vi "AlliGator Initialize Internal Variables.vi"(8 "error in (no error)":errorcluster, 9 "Alligator version":string, 10 "State Indicators":refnum<vi>, 11 "Graph References":refnum<vi>[](array[refnum])) -> (0 "error out":errorcluster, 1 "Message":string)   [LabVIEW 2021, in "AlliGator Action Engine.lvlib"]
doc: "Initializes AlliGator internal variables."
uses:
  AlliGator Action Engine.lvlib
  AlliGator State Indicators List.ctl
  Globals, Variables, Constants/AlliGator Variables List.ctl
  Image/Image Zoom Factor.ctl
  GUI/AlliGator Skippable Windows Status.ctl
  ROIs/AlliGator ROI Manager Actions.ctl
  Phasor Plot/AlliGator Phasor Harmonic Manager Actions.ctl
  Source Image/AlliGator Displayed Image.ctl
  Local Decay Window/AlliGator Local Decay Fit Results.ctl
  Image Profile Window/AlliGator Image Profile Plot Data.ctl
  Graphs/XY Graph/XY Graph Plot Data.ctl
  Image Profile Window/AlliGator Image Profile Data.ctl
  Image/Image ROI Type.ctl
  Lifetime & Other Parameters/AlliGator Lifetime & Other Parameters Plot Metadata.ctl
  GUI/AlliGator GUI.lvlib
  Globals, Variables, Constants/AlliGator Globals, Variables & Constants.lvlib
  Image/Image.lvlib
  Graphs/XY Graph/XY Graph Add-Ons.lvlib
  ROIs/AlliGator ROIs.lvlib
  Phasor Plot/AlliGator Phasor Plot.lvlib
  Image Profile Window/AlliGator Image Profile Window.lvlib
  Source Image/AlliGator Source Image.lvlib
  Local Decay Window/AlliGator Local Decay Window.lvlib
  Strings/Strings.lvlib
  Phasor Graph/AlliGator Phasor Graph.lvlib
  Lifetime & Other Parameters/AlliGator Lifetime & Other Parameters.lvlib
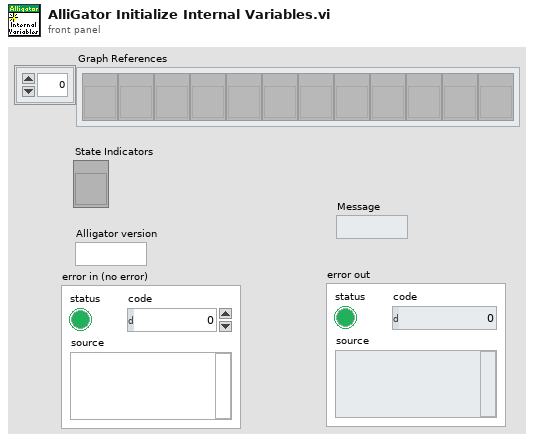
[diagram p1: front panel]
types:
  T1 = typedef "AlliGator Lifetime & Other Parameters.lvlib/AlliGator Lifetime & Other Parameters Plot Metadata.ctl" = cluster{"Intensity Array":dbl[]}
  T2 = typedef "AlliGator Image Profile Window.lvlib/AlliGator Image Profile Data.ctl" = cluster{"ROI Type":T3, "End Points":cluster{"X":dbl, "Y":dbl}[], "Profile Data":T4[]}
  T3 = typedef "Image.lvlib/Image ROI Type.ctl" = enum16{"No Selection", "Point", "Line", "Rectangle", "Oval", "Polygon", "Freehand Region", "Annulus", "Unused2", "Unused3", "Broken Line", "Freehand Line", "Rotated Rectangle"}
  T4 = typedef "AlliGator Image Profile Window.lvlib/AlliGator Image Profile Plot Data.ctl" = cluster{"Plot Name":string, "Plot":T5}
  T5 = typedef "XY Graph Add-Ons.lvlib/XY Graph Plot Data.ctl" = cluster{"X Array":dbl[], "Y Array":dbl[]}
  T6 = typedef "AlliGator Globals, Variables & Constants.lvlib/AlliGator Variables List.ctl" = enum16{"---- GUI ----", "GUI:Initialization Status", "GUI:State Indicators Refnum", "GUI:Original AlliGator Menu Items", "GUI:Current Action Loop State", "GUI:Script in progress", "GUI:Playback", "GUI:Loop Playback", "GUI:Search ROI Used", "GUI:Search ROI", "Decay Graph Max Legend Size", "Intensity Graph Max Legend Size", "Decay Statistics Graph Max Legend Size", "Phasor Graph Max Legend Size", "Phasor Ratio Graph Max Legend Size", "Lifetime Graph Max Legend Size", "---- Files ----", "Files:Export Dataset Frames as Individual Files", "Files:Show Batch Export Help Balloons", "Files:Frames in Dataset", "Files:ptu File Frame Start Indices", "Files:Current Frame in Dataset", "Files:Current Frame Timestamp", "Files:Dataset Loaded", "Files:Dataset Metadata", "Files:Dataset Channel", "Files:Dataset Data Description", "Files:Background Dataset Metadata", "Files:Background Dataset Channel", "Files:Background Dataset Data Description", "Files:Background File Subtraction", "Files:Background File Path", "Files:Background File Pile-up Correction", "Files:Background File Pixel Well Capacity", "Files:Background File Scaling Factor", "Files:Current Dataset Load Settings", "Files:Dataset Path", "Files:ICCD-specific Information", "Files:Macrotime Gate Separation", "------ Python Plugins ------", "Python Plugins:Information", "Python Plugins:Python Session", "Python Plugins:Valid Python Session?", "---- Source Image ----", "Source Image:ROIs", "Source Image:Current ROI", "Source Image:ROI Event Refnum", "X_Source Image:Display Range", "X_Source Image:Palette Information", "X_Source Image:Type of Displayed Image", "X_Time Gate Slider", "Source Image:Palette List", "Source Image:Scale", "Source Image:ROI Overlay Color", "Source Image:Overlay to Erase", "Source Image:Is Displayed Image Accumulated", "Source Image:White Light Image Modified", "Source Image:Mask Image Modified", "---- Image Profile Window ----", "Image Profile:Window Event Refnum", "Image Profile:IntensityType", "Image Profile:Intensity Average Type", "Image Profile:Intensity-weighted SDV", "Image Profile:Box Profile Type", "Image Profile:Window Open", "Image Profile:Plotted Fit Parameter", "------ Phasor Graph -------", "Phasor Graph:Show Line", "---- Phasor Plot ---", "Phasor Plot:Parameters Changed", "Phasor Plot:FLI Dataset Modified since last Calculation", "Phasor Harmonics Data", "Selected Phasor Harmonics", "Phasor Harmonic Manager Event Refnum", "Phasor Plot:ROIs", "Phasor Plot:Current ROI", "Phasor Plot:ROI Event Refnum", "Phasor Plot:Image Reference Points", "Phasor Plot:Computed", "Phasor Plot:Palette Information", "Phasor Plot:Palette List", "Phasor Plot:Phasor Ratio Palette Information", "Phasor Plot:Phasor Ratio Palette List", "Phasor Plot:Image Scale", "Phasor Plot:Image Overlay to Erase", "Phasor Plot:Image Elements to Update", "Phasor Plot:Current Calculation Parameters", "Phasor Plot:Current Calibration Options", "Phasor Plot:Reset Cumulated Phasor Plot", "Phasor Plot:Reference 1", "Phasor Plot:Lifetime Reference 1", "Phasor Plot:Reference 1 Frequency", "Phasor Plot:Reference 2", "Phasor Plot:Lifetime Reference 2", "Phasor Plot:Reference 2 Frequency", "---- Decay Analysis ----", "Number of Selected Decays to Fit", "LS Fit Results", "LAR Fit Results", "BS Fit Results", "Last Decay Max - Min", "Best Fit Parameters", "Best Fit Parameter Names", "Actual Size X", "Actual Size Y", "Binning X", "Binning Y", "Actual # Gates", "Dataset Number", "Gates to...", "Gates Skipped", "Gates to keep", "Gate Step", "Gate Separation", "Reversed Gates", "Pile-up Correction", "Pixel Well Capacity", "Background Subtracted", "Background Subtraction Method", "Background Definition Range", "Background File (deprecated)", "Number of Dataset Accumulated", "Array of Accumulated Dataset Paths", "Do Averaged Datasets", "Destination File Path", "Process Plot Target", "Use 1/D as Phasor Frequency", "---- Decay Fit Parameter Map -----", "Decay Fit Parameter Map:Palette Information", "Decay Fit Parameter Map:Palette List", "Decay Fit Parameter Map:X Resolution", "Decay Fit Parameter Map:Y Resolution", "Decay Fit Parameter Map:Use Decay Fit Result Constraints", "Decay Fit Parameter Map:Decay Fit Result Constraints", "Decay Fit Parameter Map:Decay Fit Result Constraints Applied", "---- Parameter Map ----", "Parameter Map:Palette Information", "Parameter Map:Palette List", "------- Local Decay Window ---------", "Local Decay Graph Window:Event Refnum", "Local Decay Graph Window:Use normalized IRF for convolution", "----- Miscellaneous ----", "Misc:Skippable Dialog Windows Status"}
  T7 = typedef "AlliGator Local Decay Window.lvlib/AlliGator Local Decay Fit Results.ctl" = cluster{"Decay, Fit & Residuals":T4[], "Fit Results":string}
  T8 = typedef "AlliGator Source Image.lvlib/AlliGator Displayed Image.ctl" = enum16{"Single Gate", "Sum of All Gates", "Max of All Gates", "Min of All Gates", "-", "White Ligth Image", "Mask Image"}
  T9 = typedef "AlliGator Phasor Plot.lvlib/AlliGator Phasor Harmonic Manager Actions.ctl" = enum16{"Undefined", "Delete Current Harmonic", "Delete Multiple Harmonics", "Delete All Harmonics", "Swap Harmonics", "Insert Harmonics", "Rename Current Harmonic", "Store New Harmonic", "Store Multiple Harmonics", "Select Next Harmonic", "Select Previous Harmonic", "Update Phasor Harmonic Manager Window"}
  T10 = typedef "AlliGator ROIs.lvlib/AlliGator ROI Manager Actions.ctl" = enum16{"Undefined", "Delete Current ROI", "Delete All Unselected ROIs", "Delete Multiple ROIs", "Delete All ROIs", "Swap ROIs", "Insert ROI", "Update Current ROI Descriptor", "Rename Current ROI", "Store New ROI", "Store Multiple ROIs", "Select Next ROI", "Select Previous ROI", "Find Selected ROI", "Show All ROIs", "Update ROI Manager Window", "Merge All ROIs", "Unmerge ROI", "Set Selected ROI by ID"}
  T11 = typedef "AlliGator GUI.lvlib/AlliGator Skippable Windows Status.ctl" = cluster{"Dialog Window Name":string, "Is skipped":bool}
  T12 = typedef "Image.lvlib/Image Zoom Factor.ctl" = enum16{"Zoom to Fit", "Zoom to Fit (Keep Aspect Ratio)", "Other Zoom Factor"}
  T13 = typedef "AlliGator Action Engine.lvlib/AlliGator State Indicators List.ctl" = enum16{"Phasor Calibration Defined", "Phasor Calibration Series Defined", "Phasor Calibration Map Defined", "Phasor Reference 1 Defined", "Phasor Reference 2 Defined", "Lifetime Reference 1 Defined", "Lifetime Reference 2 Defined", "Phasor Calibration Used", "Phasor Calibration Series Used", "Phasor Calibration Map Used", "Dataset Update Needed", "Phasor Plot Update Needed", "Reference/IRF Defined", "Individual IRFs Defined"}
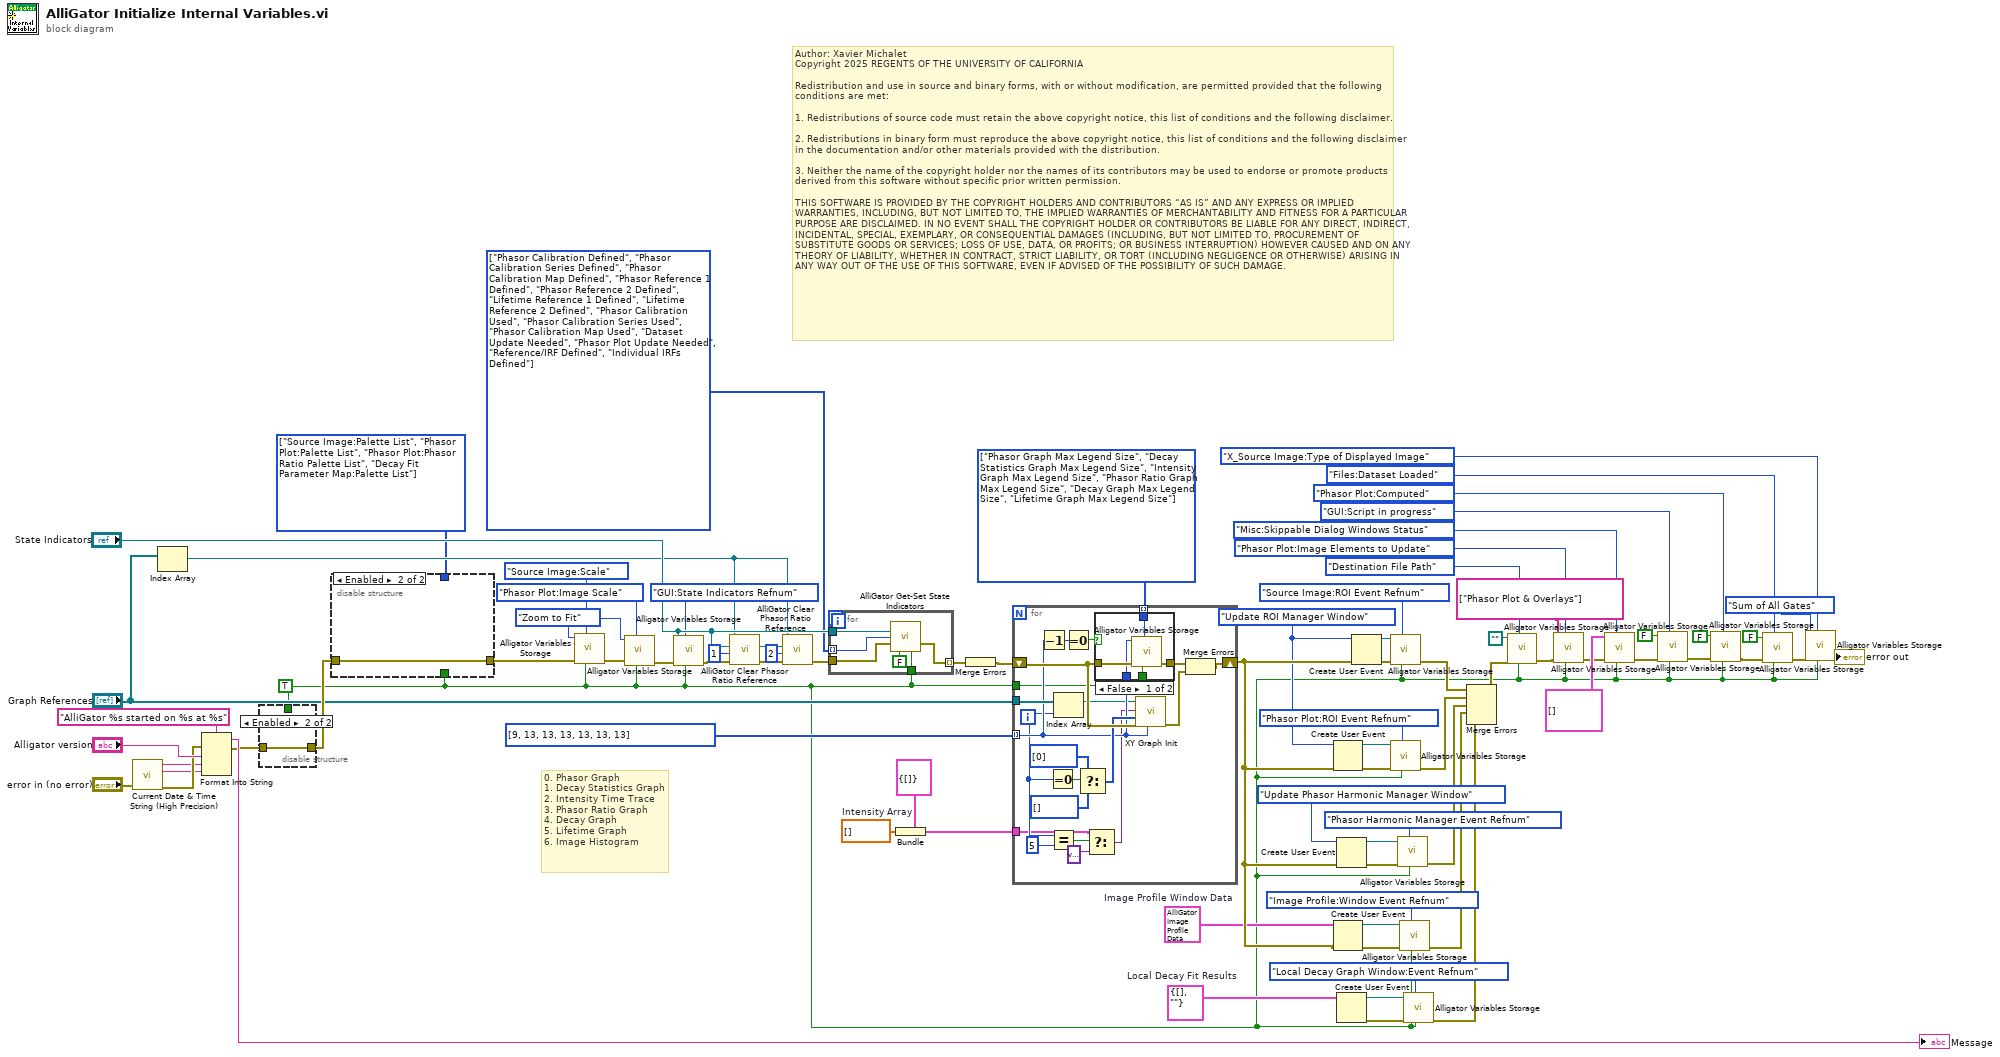
[diagram p0: block diagram]
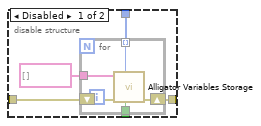
[diagram p2: hidden frame]
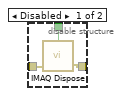
[diagram p3: hidden frame]
diagram:
  w3 = dbl[] []  # Intensity Array
  w6 = T2 {"ROI Type"=enum."No Selection", "End Points"=[{"X"=98.0, "Y"=43.0}, {"X"=133.0, "Y"=78.0}], "Profile Data"=[]}  # Image Profile Window Data
  w8 = T6[] [enum."Source Image:Palette List", enum."Phasor Plot:Palette List", enum."Phasor Plot:Phasor Ratio Palette List", enum."Decay Fit Parameter Map:Palette List"] items=["---- GUI ----", "GUI:Initialization Status", "GUI:State Indicators Refnum", "GUI:Original AlliGator Menu Items", "GUI:Current Action Loop State", "GUI:Script in progress", "GUI:Playback", "GUI:Loop Playback", "GUI:Search ROI Used", "GUI:Search ROI", "Decay Graph Max Legend Size", "Intensity Graph Max Legend Size", "Decay Statistics Graph Max Legend Size", "Phasor Graph Max Legend Size", "Phasor Ratio Graph Max Legend Size", "Lifetime Graph Max Legend Size", "---- Files ----", "Files:Export Dataset Frames as Individual Files", "Files:Show Batch Export Help Balloons", "Files:Frames in Dataset", "Files:ptu File Frame Start Indices", "Files:Current Frame in Dataset", "Files:Current Frame Timestamp", "Files:Dataset Loaded", "Files:Dataset Metadata", "Files:Dataset Channel", "Files:Dataset Data Description", "Files:Background Dataset Metadata", "Files:Background Dataset Channel", "Files:Background Dataset Data Description", "Files:Background File Subtraction", "Files:Background File Path", "Files:Background File Pile-up Correction", "Files:Background File Pixel Well Capacity", "Files:Background File Scaling Factor", "Files:Current Dataset Load Settings", "Files:Dataset Path", "Files:ICCD-specific Information", "Files:Macrotime Gate Separation", "------ Python Plugins ------", "Python Plugins:Information", "Python Plugins:Python Session", "Python Plugins:Valid Python Session?", "---- Source Image ----", "Source Image:ROIs", "Source Image:Current ROI", "Source Image:ROI Event Refnum", "X_Source Image:Display Range", "X_Source Image:Palette Information", "X_Source Image:Type of Displayed Image", "X_Time Gate Slider", "Source Image:Palette List", "Source Image:Scale", "Source Image:ROI Overlay Color", "Source Image:Overlay to Erase", "Source Image:Is Displayed Image Accumulated", "Source Image:White Light Image Modified", "Source Image:Mask Image Modified", "---- Image Profile Window ----", "Image Profile:Window Event Refnum", "Image Profile:IntensityType", "Image Profile:Intensity Average Type", "Image Profile:Intensity-weighted SDV", "Image Profile:Box Profile Type", "Image Profile:Window Open", "Image Profile:Plotted Fit Parameter", "------ Phasor Graph -------", "Phasor Graph:Show Line", "---- Phasor Plot ---", "Phasor Plot:Parameters Changed", "Phasor Plot:FLI Dataset Modified since last Calculation", "Phasor Harmonics Data", "Selected Phasor Harmonics", "Phasor Harmonic Manager Event Refnum", "Phasor Plot:ROIs", "Phasor Plot:Current ROI", "Phasor Plot:ROI Event Refnum", "Phasor Plot:Image Reference Points", "Phasor Plot:Computed", "Phasor Plot:Palette Information", "Phasor Plot:Palette List", "Phasor Plot:Phasor Ratio Palette Information", "Phasor Plot:Phasor Ratio Palette List", "Phasor Plot:Image Scale", "Phasor Plot:Image Overlay to Erase", "Phasor Plot:Image Elements to Update", "Phasor Plot:Current Calculation Parameters", "Phasor Plot:Current Calibration Options", "Phasor Plot:Reset Cumulated Phasor Plot", "Phasor Plot:Reference 1", "Phasor Plot:Lifetime Reference 1", "Phasor Plot:Reference 1 Frequency", "Phasor Plot:Reference 2", "Phasor Plot:Lifetime Reference 2", "Phasor Plot:Reference 2 Frequency", "---- Decay Analysis ----", "Number of Selected Decays to Fit", "LS Fit Results", "LAR Fit Results", "BS Fit Results", "Last Decay Max - Min", "Best Fit Parameters", "Best Fit Parameter Names", "Actual Size X", "Actual Size Y", "Binning X", "Binning Y", "Actual # Gates", "Dataset Number", "Gates to...", "Gates Skipped", "Gates to keep", "Gate Step", "Gate Separation", "Reversed Gates", "Pile-up Correction", "Pixel Well Capacity", "Background Subtracted", "Background Subtraction Method", "Background Definition Range", "Background File (deprecated)", "Number of Dataset Accumulated", "Array of Accumulated Dataset Paths", "Do Averaged Datasets", "Destination File Path", "Process Plot Target", "Use 1/D as Phasor Frequency", "---- Decay Fit Parameter Map -----", "Decay Fit Parameter Map:Palette Information", "Decay Fit Parameter Map:Palette List", "Decay Fit Parameter Map:X Resolution", "Decay Fit Parameter Map:Y Resolution", "Decay Fit Parameter Map:Use Decay Fit Result Constraints", "Decay Fit Parameter Map:Decay Fit Result Constraints", "Decay Fit Parameter Map:Decay Fit Result Constraints Applied", "---- Parameter Map ----", "Parameter Map:Palette Information", "Parameter Map:Palette List", "------- Local Decay Window ---------", "Local Decay Graph Window:Event Refnum", "Local Decay Graph Window:Use normalized IRF for convolution", "----- Miscellaneous ----", "Misc:Skippable Dialog Windows Status"] ("Array")
  w67 = T7 {"Decay, Fit & Residuals"=[], "Fit Results"=""}  # Local Decay Fit Results
  w49 = AlliGator_ROI_Manager_Actions."Update ROI Manager Window" ("Action")
  w20 = T6[] [enum."Phasor Graph Max Legend Size", enum."Decay Statistics Graph Max Legend Size", enum."Intensity Graph Max Legend Size", enum."Phasor Ratio Graph Max Legend Size", enum."Decay Graph Max Legend Size", enum."Lifetime Graph Max Legend Size"] items=["---- GUI ----", "GUI:Initialization Status", "GUI:State Indicators Refnum", "GUI:Original AlliGator Menu Items", "GUI:Current Action Loop State", "GUI:Script in progress", "GUI:Playback", "GUI:Loop Playback", "GUI:Search ROI Used", "GUI:Search ROI", "Decay Graph Max Legend Size", "Intensity Graph Max Legend Size", "Decay Statistics Graph Max Legend Size", "Phasor Graph Max Legend Size", "Phasor Ratio Graph Max Legend Size", "Lifetime Graph Max Legend Size", "---- Files ----", "Files:Export Dataset Frames as Individual Files", "Files:Show Batch Export Help Balloons", "Files:Frames in Dataset", "Files:ptu File Frame Start Indices", "Files:Current Frame in Dataset", "Files:Current Frame Timestamp", "Files:Dataset Loaded", "Files:Dataset Metadata", "Files:Dataset Channel", "Files:Dataset Data Description", "Files:Background Dataset Metadata", "Files:Background Dataset Channel", "Files:Background Dataset Data Description", "Files:Background File Subtraction", "Files:Background File Path", "Files:Background File Pile-up Correction", "Files:Background File Pixel Well Capacity", "Files:Background File Scaling Factor", "Files:Current Dataset Load Settings", "Files:Dataset Path", "Files:ICCD-specific Information", "Files:Macrotime Gate Separation", "------ Python Plugins ------", "Python Plugins:Information", "Python Plugins:Python Session", "Python Plugins:Valid Python Session?", "---- Source Image ----", "Source Image:ROIs", "Source Image:Current ROI", "Source Image:ROI Event Refnum", "X_Source Image:Display Range", "X_Source Image:Palette Information", "X_Source Image:Type of Displayed Image", "X_Time Gate Slider", "Source Image:Palette List", "Source Image:Scale", "Source Image:ROI Overlay Color", "Source Image:Overlay to Erase", "Source Image:Is Displayed Image Accumulated", "Source Image:White Light Image Modified", "Source Image:Mask Image Modified", "---- Image Profile Window ----", "Image Profile:Window Event Refnum", "Image Profile:IntensityType", "Image Profile:Intensity Average Type", "Image Profile:Intensity-weighted SDV", "Image Profile:Box Profile Type", "Image Profile:Window Open", "Image Profile:Plotted Fit Parameter", "------ Phasor Graph -------", "Phasor Graph:Show Line", "---- Phasor Plot ---", "Phasor Plot:Parameters Changed", "Phasor Plot:FLI Dataset Modified since last Calculation", "Phasor Harmonics Data", "Selected Phasor Harmonics", "Phasor Harmonic Manager Event Refnum", "Phasor Plot:ROIs", "Phasor Plot:Current ROI", "Phasor Plot:ROI Event Refnum", "Phasor Plot:Image Reference Points", "Phasor Plot:Computed", "Phasor Plot:Palette Information", "Phasor Plot:Palette List", "Phasor Plot:Phasor Ratio Palette Information", "Phasor Plot:Phasor Ratio Palette List", "Phasor Plot:Image Scale", "Phasor Plot:Image Overlay to Erase", "Phasor Plot:Image Elements to Update", "Phasor Plot:Current Calculation Parameters", "Phasor Plot:Current Calibration Options", "Phasor Plot:Reset Cumulated Phasor Plot", "Phasor Plot:Reference 1", "Phasor Plot:Lifetime Reference 1", "Phasor Plot:Reference 1 Frequency", "Phasor Plot:Reference 2", "Phasor Plot:Lifetime Reference 2", "Phasor Plot:Reference 2 Frequency", "---- Decay Analysis ----", "Number of Selected Decays to Fit", "LS Fit Results", "LAR Fit Results", "BS Fit Results", "Last Decay Max - Min", "Best Fit Parameters", "Best Fit Parameter Names", "Actual Size X", "Actual Size Y", "Binning X", "Binning Y", "Actual # Gates", "Dataset Number", "Gates to...", "Gates Skipped", "Gates to keep", "Gate Step", "Gate Separation", "Reversed Gates", "Pile-up Correction", "Pixel Well Capacity", "Background Subtracted", "Background Subtraction Method", "Background Definition Range", "Background File (deprecated)", "Number of Dataset Accumulated", "Array of Accumulated Dataset Paths", "Do Averaged Datasets", "Destination File Path", "Process Plot Target", "Use 1/D as Phasor Frequency", "---- Decay Fit Parameter Map -----", "Decay Fit Parameter Map:Palette Information", "Decay Fit Parameter Map:Palette List", "Decay Fit Parameter Map:X Resolution", "Decay Fit Parameter Map:Y Resolution", "Decay Fit Parameter Map:Use Decay Fit Result Constraints", "Decay Fit Parameter Map:Decay Fit Result Constraints", "Decay Fit Parameter Map:Decay Fit Result Constraints Applied", "---- Parameter Map ----", "Parameter Map:Palette Information", "Parameter Map:Palette List", "------- Local Decay Window ---------", "Local Decay Graph Window:Event Refnum", "Local Decay Graph Window:Use normalized IRF for convolution", "----- Miscellaneous ----", "Misc:Skippable Dialog Windows Status"] ("Array")
  w18 = Image_Zoom_Factor."Zoom to Fit" ("Image Zoom Factor")
  w5 = TRUE ("Get(F)/Set")
  w15 = T13[] [enum."Phasor Calibration Defined", enum."Phasor Calibration Series Defined", enum."Phasor Calibration Map Defined", enum."Phasor Reference 1 Defined", enum."Phasor Reference 2 Defined", enum."Lifetime Reference 1 Defined", enum."Lifetime Reference 2 Defined", enum."Phasor Calibration Used", enum."Phasor Calibration Series Used", enum."Phasor Calibration Map Used", enum."Dataset Update Needed", enum."Phasor Plot Update Needed", enum."Reference/IRF Defined", enum."Individual IRFs Defined"] items=["Phasor Calibration Defined", "Phasor Calibration Series Defined", "Phasor Calibration Map Defined", "Phasor Reference 1 Defined", "Phasor Reference 2 Defined", "Lifetime Reference 1 Defined", "Lifetime Reference 2 Defined", "Phasor Calibration Used", "Phasor Calibration Series Used", "Phasor Calibration Map Used", "Dataset Update Needed", "Phasor Plot Update Needed", "Reference/IRF Defined", "Individual IRFs Defined"] ("Array")
  # "Author: Xavier Michalet\nCopyright 2025 REGENTS OF THE UNIVERSITY OF CALIFORNIA\n\nRedistribution and use in source and binary forms, with or without modification, are permitted provided that the following conditions are met:\n\n1. Redistributions of source code must retain the above copyright notice, this list of conditions and the following disclaimer.\n\n2. Redistributions in binary form must reproduce the above copyright notice, this list of conditions and the following disclaimer in the documentation and/or other materials provided with the distribution.\n\n3. Neither the name of the copyright holder nor the names of its contributors may be used to endorse or promote products derived from this software without specific prior written permission.\n\nTHIS SOFTWARE IS PROVIDED BY THE COPYRIGHT HOLDERS AND CONTRIBUTORS “AS IS” AND ANY EXPRESS OR IMPLIED WARRANTIES, INCLUDING, BUT NOT LIMITED TO, THE IMPLIED WARRANTIES OF MERCHANTABILITY AND FITNESS FOR A PARTICULAR PURPOSE ARE DISCLAIMED. IN NO EVENT SHALL THE COPYRIGHT HOLDER OR CONTRIBUTORS BE LIABLE FOR ANY DIRECT, INDIRECT, INCIDENTAL, SPECIAL, EXEMPLARY, OR CONSEQUENTIAL DAMAGES (INCLUDING, BUT NOT LIMITED TO, PROCUREMENT OF SUBSTITUTE GOODS OR SERVICES; LOSS OF USE, DATA, OR PROFITS; OR BUSINESS INTERRUPTION) HOWEVER CAUSED AND ON ANY THEORY OF LIABILITY, WHETHER IN CONTRACT, STRICT LIABILITY, OR TORT (INCLUDING NEGLIGENCE OR OTHERWISE) ARISING IN ANY WAY OUT OF THE USE OF THIS SOFTWARE, EVEN IF ADVISED OF THE POSSIBILITY OF SUCH DAMAGE."
  # "0. Phasor Graph\n1. Decay Statistics Graph\n2. Intensity Time Trace\n3. Phasor Ratio Graph\n4. Decay Graph\n5. Lifetime Graph\n6. Image Histogram"
  n1 = call "Current Date & Time String (High Precision).vi"("Error In"="error in (no error)") -> ("Error Out"=w73:errorcluster, "time string"=w72:string, "date string"=w71:string)  [unwired: 7 in, 1 out]
  n2 = Index Array(array="Graph References") -> (element=w13:refnum<vi>)  [unwired: 1 in]
  n3 = Format Into String(format string="AlliGator %s started on %s at %s" ("initial string"), error in=w73, "Alligator version", w71, w72) -> (resulting string=→"Message":string, error out=w9:errorcluster)  [unwired: 1 in]
  n4 = disable-structure shown="Enabled" {
    disable-tunnel: [w84 w85] -> w80
    disable-tunnel: w5 -> [w83 _]
    disable-tunnel: w9 -> [w82 w85]
    frame Disabled {
      n5 = call "IMAQ Dispose"("All Images? (No)"=w83, "error in (no error)"=w82) -> ("error out"=w84:errorcluster)  [unwired: 4 in]
    }
    frame Enabled {
    }
  }
  n6 = disable-structure shown="Enabled" {
    disable-tunnel: w5 -> [w90 _]
    disable-tunnel: w80 -> [w89 w96]
    disable-tunnel: w8 -> [w87 _]
    disable-tunnel: [w86 w96] -> w7
    frame Disabled {
      n7 = for {
        tunnel: w90 -> [w95]
        tunnel: string[] [] ("String Array") -> [w93]
        tunnel: w87 -> [w92] mode=indexing
        shift-right: [w91] -> w86
        shift-left: w89 -> [w94]
        n8 = call "Alligator Variables Storage.vi"("Get(F)/Set"=w95, "AlliGator Variable"=w92, "Error In"=w94, "Data in"=w93) -> ("Error Out"=w91:errorcluster)  [unwired: 5 in, 2 out]
      }
    }
    frame Enabled {
    }
  }
  n9 = call "Alligator Variables Storage.vi"("Get(F)/Set"=w5, "AlliGator Variable"=AlliGator_Variables_List."Source Image:Scale" ("Alligator Variable"), "Error In"=w7, "Data in"=w18) -> ("Error Out"=w17:errorcluster)  [unwired: 5 in, 2 out]
  n10 = call "Alligator Variables Storage.vi"("Get(F)/Set"=w5, "AlliGator Variable"=AlliGator_Variables_List."Phasor Plot:Image Scale" ("Alligator Variable"), "Error In"=w17, "Data in"=w18) -> ("Error Out"=w81:errorcluster)  [unwired: 5 in, 2 out]
  n11 = call "Alligator Variables Storage.vi"("Get(F)/Set"=w5, "AlliGator Variable"=AlliGator_Variables_List."GUI:State Indicators Refnum" ("Alligator Variable"), "Error In"=w81, "Data in"="State Indicators") -> ("Error Out"=w75:errorcluster)  [unwired: 5 in, 2 out]
  n12 = call "AlliGator Clear Phasor Ratio Reference.vi"("error in (no error)"=w75, "Reference Number"=1, "State Indicators Refnum"="State Indicators", "Phasor Graph Refnum"=w13) -> ("Error Out"=w76:errorcluster)  [unwired: 7 in]
  n13 = call "AlliGator Clear Phasor Ratio Reference.vi"("error in (no error)"=w76, "Reference Number"=2, "State Indicators Refnum"="State Indicators", "Phasor Graph Refnum"=w13) -> ("Error Out"=w11:errorcluster)  [unwired: 7 in]
  n14 = for {
    tunnel: "State Indicators" -> [w102]
    tunnel: w15 -> [w101] mode=indexing
    tunnel: w11 -> [w99]
    tunnel: [w98] -> w68 mode=indexing
    tunnel: w5 -> [w97]
    n15 = call "AlliGator Get-Set State Indicators.vi"("State Indicators Refnum"=w102, "AlliGator State Indicators List"=w101, "Error In"=w99, "ON/OFF"=FALSE ("Set (T)/Unset (F)"), "Set (T)/Get"=w97) -> ("Error Out"=w98:errorcluster)  [unwired: 8 in, 2 out]
  }
  n16 = Bundle(cluster=T1 {"Intensity Array"=[]}, "Intensity Array"=w3) -> (w2:T1)
  n17 = Merge Errors(w68) -> (w12:errorcluster)
  n18 = for {
    tunnel: w20 -> [w123] mode=indexing
    tunnel: w5 -> [w109]
    shift-right: [w119] -> w58
    shift-left: w12 -> [w120]
    tunnel: i32[] [9, 13, 13, 13, 13, 13, 13] ("Max Legend Size (8)") -> [w113] mode=indexing
    tunnel: "Graph References" -> [w121]
    tunnel: w2 -> [w105]
    i -> [w108]
    n19 = Decrement(x=w113) -> (x-1=w112:i32)
    n20 = Equal To 0?(x=w108) -> (x = 0?=w117:bool)
    n21 = Equal?(x=w108, y=5) -> (x = y?=w106:bool)
    n22 = Index Array(array=w121, index=w108) -> (element=w110:refnum<vi>)
    n23 = Equal To 0?(x=w112) -> (x = 0?=w111:bool)
    n24 = Select(t=i32[] [0] ("Plots to Skip (none)"), s=w117, f=i32[] []) -> (s? t:f=w116:i32[])
    n25 = Select(t=w105, s=w106, f=variant) -> (s? t:f=w103:variant)
    n26 = case shown="False" w111 {
      tunnel: w123 -> [w128 _]
      tunnel: [w127 w129] -> w122
      tunnel: w120 -> [w126 w129]
      tunnel: w113 -> [w125 _]
      tunnel: w109 -> [w124 _]
      frame False {
        n27 = call "Alligator Variables Storage.vi"("Get(F)/Set"=w124, "AlliGator Variable"=w128, "Error In"=w126, "Data in"=w125) -> ("Error Out"=w127:errorcluster)  [unwired: 5 in, 2 out]
      }
      frame True {
      }
    }
    n28 = call "XY Graph Init.vi"("Max Legend Size (8)"=w113, "Error In"=w120, "Plots to Skip (none)"=w116, "Metadata Type"=w103, "XYGraph in"=w110) -> ("Error Out"=w118:errorcluster)  [unwired: 6 in]
    n29 = Merge Errors(w122, w118) -> (w119:errorcluster)
  }
  n30 = Create User Event(user event datatype=w49, error in=w58) -> (user event=w45:refnum<user-event>, error out=w44:errorcluster)
  n31 = Create User Event(user event datatype=w6, error in=w58) -> (user event=w4:refnum<user-event>, error out=w55:errorcluster)
  n32 = Create User Event(user event datatype=AlliGator_Phasor_Harmonic_Manager_Actions."Update Phasor Harmonic Manager Window" ("Action"), error in=w58) -> (user event=w52:refnum<user-event>, error out=w51:errorcluster)
  n33 = Create User Event(user event datatype=w67) -> (user event=w64:refnum<user-event>, error out=w65:errorcluster)  [unwired: 1 in]
  n34 = Create User Event(user event datatype=w49, error in=w58) -> (user event=w22:refnum<user-event>, error out=w23:errorcluster)
  n35 = call "Alligator Variables Storage.vi"("Get(F)/Set"=w5, "AlliGator Variable"=AlliGator_Variables_List."Source Image:ROI Event Refnum" ("Alligator Variable"), "Error In"=w23, "Data in"=w22) -> ("Error Out"=w24:errorcluster)  [unwired: 5 in, 2 out]
  n36 = call "Alligator Variables Storage.vi"("Get(F)/Set"=w5, "AlliGator Variable"=AlliGator_Variables_List."Phasor Plot:ROI Event Refnum" ("Alligator Variable"), "Error In"=w44, "Data in"=w45) -> ("Error Out"=w47:errorcluster)  [unwired: 5 in, 2 out]
  n37 = call "Alligator Variables Storage.vi"("Get(F)/Set"=w5, "AlliGator Variable"=AlliGator_Variables_List."Phasor Harmonic Manager Event Refnum" ("Alligator Variable"), "Error In"=w51, "Data in"=w52) -> ("Error Out"=w53:errorcluster)  [unwired: 5 in, 2 out]
  n38 = call "Alligator Variables Storage.vi"("Get(F)/Set"=w5, "AlliGator Variable"=AlliGator_Variables_List."Image Profile:Window Event Refnum" ("Alligator Variable"), "Error In"=w55, "Data in"=w4) -> ("Error Out"=w57:errorcluster)  [unwired: 5 in, 2 out]
  n39 = call "Alligator Variables Storage.vi"("Get(F)/Set"=w5, "AlliGator Variable"=AlliGator_Variables_List."Local Decay Graph Window:Event Refnum" ("Alligator Variable"), "Error In"=w65, "Data in"=w64) -> ("Error Out"=w66:errorcluster)  [unwired: 5 in, 2 out]
  n40 = Merge Errors(w24, w47, w53, w57, w66) -> (w46:errorcluster)
  n41 = call "Alligator Variables Storage.vi"("Get(F)/Set"=w5, "AlliGator Variable"=AlliGator_Variables_List."Destination File Path" ("Alligator Variable"), "Error In"=w46, "Data in"=path "") -> ("Error Out"=w27:errorcluster)  [unwired: 5 in, 2 out]
  n42 = call "Alligator Variables Storage.vi"("Get(F)/Set"=w5, "AlliGator Variable"=AlliGator_Variables_List."Phasor Plot:Image Elements to Update" ("Alligator Variable"), "Error In"=w27, "Data in"=string[] ["Phasor Plot & Overlays"] ("element")) -> ("Error Out"=w31:errorcluster)  [unwired: 5 in, 2 out]
  n43 = call "Alligator Variables Storage.vi"("Get(F)/Set"=w5, "AlliGator Variable"=AlliGator_Variables_List."Misc:Skippable Dialog Windows Status" ("Alligator Variable"), "Error In"=w31, "Data in"=T11[] []) -> ("Error Out"=w34:errorcluster)  [unwired: 5 in, 2 out]
  n44 = call "Alligator Variables Storage.vi"("Get(F)/Set"=w5, "AlliGator Variable"=AlliGator_Variables_List."GUI:Script in progress" ("Alligator Variable"), "Error In"=w34, "Data in"=FALSE ("Get(F)/Set")) -> ("Error Out"=w38:errorcluster)  [unwired: 5 in, 2 out]
  n45 = call "Alligator Variables Storage.vi"("Get(F)/Set"=w5, "AlliGator Variable"=AlliGator_Variables_List."Phasor Plot:Computed" ("Alligator Variable"), "Error In"=w38, "Data in"=FALSE ("Set (T)/Unset (F)")) -> ("Error Out"=w41:errorcluster)  [unwired: 5 in, 2 out]
  n46 = call "Alligator Variables Storage.vi"("Get(F)/Set"=w5, "AlliGator Variable"=AlliGator_Variables_List."Files:Dataset Loaded" ("Alligator Variable"), "Error In"=w41, "Data in"=FALSE ("Set (T)/Unset (F)")) -> ("Error Out"=w59:errorcluster)  [unwired: 5 in, 2 out]
  n47 = call "Alligator Variables Storage.vi"("Get(F)/Set"=w5, "AlliGator Variable"=AlliGator_Variables_List."X_Source Image:Type of Displayed Image" ("Alligator Variable"), "Error In"=w59, "Data in"=AlliGator_Displayed_Image."Sum of All Gates" ("Displayed Image")) -> ("Error Out"=→"error out":errorcluster)  [unwired: 5 in, 2 out]
